vi "Read Shutter Open_.vi"(8 "error in (no error)":errorcluster, 11 "Spectrometer Triax 550 in":refnum<class "Spectrometer Triax 550.lvclass">) -> (0 "error out":errorcluster, 2 "Shutter Open?":bool, 3 "Spectrometer Triax 550 out":refnum<class "Spectrometer Triax 550.lvclass">)   [LabVIEW 2017, in "Spectrometer Triax 550.lvclass"]
uses:
  Spectrometer Triax 550.lvclass
  Spectrometer Triax 550.lvclass/Spectrometer Triax 550.ctl
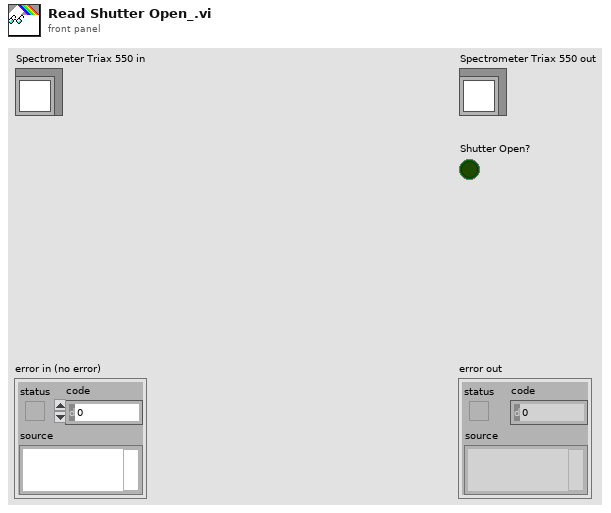
[diagram p1: front panel]
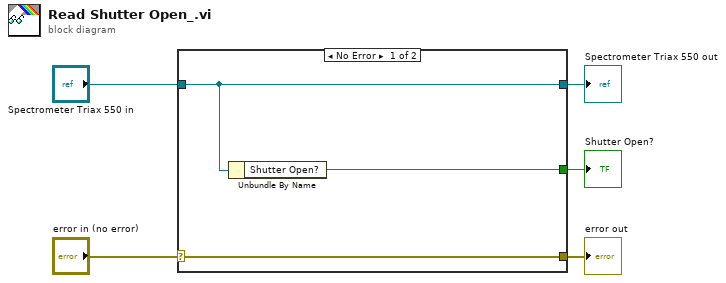
[diagram p0: block diagram]
diagram:
  n1 = case shown="No Error" "error in (no error)" {
    selector: "error in (no error)" -> [w8 w9]
    tunnel: [w8 w9] -> w4
    tunnel: [w7 w10] -> w2
    tunnel: "Spectrometer Triax 550 in" -> [w7 w10]
    tunnel: [w6 _] -> w1
    frame No Error {
      n2 = Unbundle By Name(w7) -> ("Shutter Open?"=w6:bool)
    }
    frame Error {
    }
  }
  "error out" <- w4
  "Spectrometer Triax 550 out" <- w2
  "Shutter Open?" <- w1
